vi "Create Mappings.vi"(10 "Lines":T1[](array[typedef]), 11 "data allocations":T2) -> (0 "Output Mapping":T5[](array[typedef]), 1 "Input Mapping":T5[](array[typedef]), 2 "Output Singals":refnum<k21>[](array[refnum]), 3 "Input Singals":refnum<k21>[](array[refnum]))   [LabVIEW 2013, in "J1939 runtime.lvclass"]
uses:
  J1939 runtime.lvclass
  configuration/Signal Mapping.ctl
  <vilib>/NI/Tag Bus/tag/Data Type.ctl
  <vilib>/NI/Tag Bus Module Framework/channel/data tables.ctl
  <vilib>/NI/Tag Bus/dictionary/data dictionary.lvclass
  <vilib>/NI/Tag Bus/dictionary table pair.ctl
  <vilib>/NI/Tag Bus/table/data table.ctl
  configuration/Line.ctl
  <vilib>/NI/Tag Bus Module Framework/channel/TBM channel.lvclass
  <vilib>/NI/Tag Bus Module Framework/channel/channel classification.ctl
  <vilib>/NI/Tag Bus Module Framework/channel/TBM channel.lvclass/TBM channel.ctl
  <vilib>/NI/Tag Bus/tag/tag descriptor.lvclass
  configuration/J1939 configuration.lvclass
  <vilib>/NI/Tag Bus/table/data table.lvlib
  <vilib>/NI/Tag Bus/tag bus.lvlib
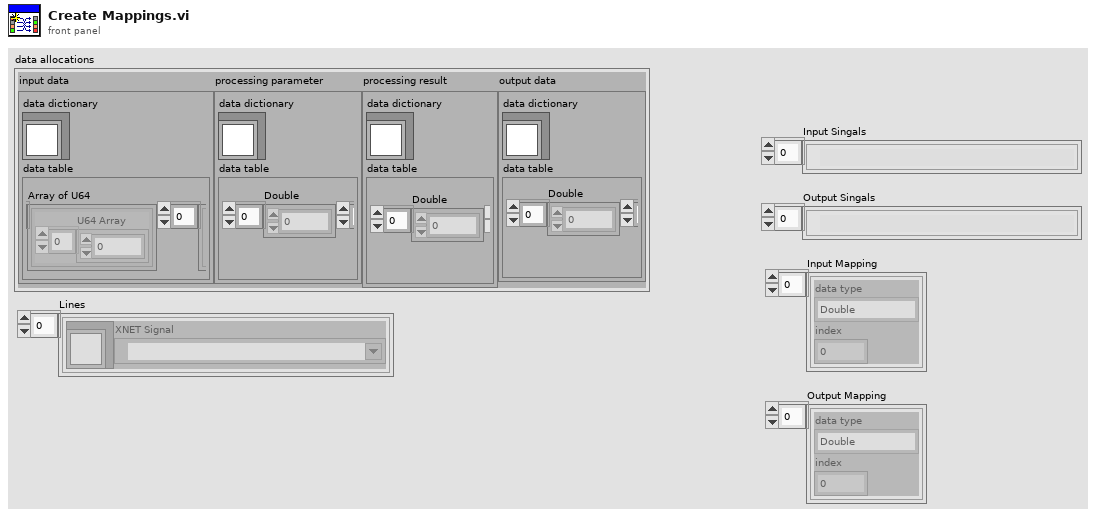
[diagram p1: front panel]
types:
  T1 = typedef "J1939 configuration.lvclass/Line.ctl" = cluster{"channel":refnum<class "TBM channel.lvclass">, "XNET Signal":refnum<k21>}
  T2 = typedef "TBM channel.lvclass/data tables.ctl" = cluster{"input data":T3, "processing parameter":T3, "processing result":T3, "output data":T3}
  T3 = typedef "tag bus.lvlib/dictionary table pair.ctl" = cluster{"data dictionary":refnum<class "data dictionary.lvclass">, "data table":T4}
  T4 = typedef "tag bus.lvlib/data table.lvlib/data table.ctl" = cluster{"Double":dbl[], "Single":sgl[], "I64":i64[], "I32":i32[], "I16":i16[], "I8":i8[], "U64":u64[], "U32":u32[], "U16":u16[], "U8":u8[], "Boolean":bool[], "String":string[], "Array of Double":cluster{"DBL Array":dbl[]}[], "Array of Single":cluster{"SGL Array":sgl[]}[], "Array of I64":cluster{"I64 Array":i64[]}[], "Array of I32":cluster{"I32 Array":i32[]}[], "Array of I16":cluster{"I16 Array":i16[]}[], "Array of I8":cluster{"I8 Array":i8[]}[], "Array of U64":cluster{"U64 Array":u64[]}[], "Array of U32":cluster{"U32 Array":u32[]}[], "Array of U16":cluster{"U16 Array":u16[]}[], "Array of U8":cluster{"U8 Array":u8[]}[], "Array of Boolean":cluster{"Boolean Array":bool[]}[], "Array of String":cluster{"String Array":string[]}[]}
  T5 = typedef "J1939 configuration.lvclass/Signal Mapping.ctl" = cluster{"data type":T6, "index":i32}
  T6 = typedef "tag bus.lvlib/tag descriptor.lvclass/Data Type.ctl" = enum16{"Double", "Single", "I64", "I32", "I16", "I8", "U64", "U32", "U16", "U8", "Boolean", "String", "Array of Double", "Array of Single", "Array of I64", "Array of I32", "Array of I16", "Array of I8", "Array of U64", "Array of U32", "Array of U16", "Array of U8", "Array of Boolean", "Array of String"}
  T7 = typedef "TBM channel.lvclass/channel classification.ctl" = enum16{"input data", "output data", "processing parameter", "processing result"}
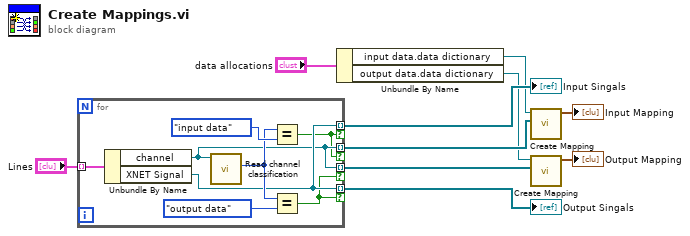
[diagram p0: block diagram]
diagram:
  n1 = for {
    tunnel: "Lines" -> [w18] mode=indexing
    tunnel: [w14] -> w8 mode=indexing if=w12
    tunnel: [w14] -> w9 mode=indexing if=w11
    tunnel: [w13] -> w5 mode=indexing if=w12
    tunnel: [w13] -> w3 mode=indexing if=w11
    n2 = Unbundle By Name(w18) -> ("channel"=w13:refnum<class "TBM channel.lvclass">, "XNET Signal"=w14:refnum<k21>)
    n3 = call <vilib>:"Read channel classification.vi"("channel in"=w13) -> ("channel classification"=w16:T7)  [unwired: 8 in, 2 out]
    n4 = Equal?(x=w16, y=channel_classification."input data") -> (x = y?=w12:bool)
    n5 = Equal?(x=w16, y=channel_classification."output data") -> (x = y?=w11:bool)
  }
  "Output Singals" <- w9
  "Input Singals" <- w8
  n6 = Unbundle By Name("data allocations") -> ("input data.data dictionary"=w6:refnum<class "data dictionary.lvclass">, "output data.data dictionary"=w4:refnum<class "data dictionary.lvclass">)
  n7 = call "Create Mapping.vi"("Channels In"=w5, "Data Dictionary In"=w6) -> ("Array out"=→"Input Mapping":T5[])  [unwired: 9 in]
  n8 = call "Create Mapping.vi"("Channels In"=w3, "Data Dictionary In"=w4) -> ("Array out"=→"Output Mapping":T5[])  [unwired: 9 in]
